vi "Leakage_Keithley6517A.vi"(5 "Number of Points":sgl=1.0 min=0 max=9999.9 step=0.1 format="%.1f", 6 "Interval(secs)":sgl=1.0 min=0 max=9999.9 step=0.1 format="%.1f", 7 "Bias Voltage":sgl=1.0 min=-1000 max=1000 step=0.1 format="%.1f", 8 "error in":T1, 11 "GPIB address":string="27") -> (0 "error out":T1, 3 "Test Data":sgl[][](array[numeric])=[[1.0, 2.2355776e-13]] format="%.6p")   [LabVIEW 2010]
doc: "This VI performs the Capacitor Leakage Test Sequence in the 6517A. \n\nParameters:\nGPIB Address: Default to 27\n\nBias Voltage\n-1000 to +1000\n\nBias Time:\n0 to 9999.9\n\nDischarge Time:\n0 to 9999.9"
panel:
  in  "control":sgl[](array[numeric]) format="%.2f"
  out "?":string="Current"
  # "KEITHLEY"
  # "6517A Capacitor Leakage Test"
  # "Voltage"
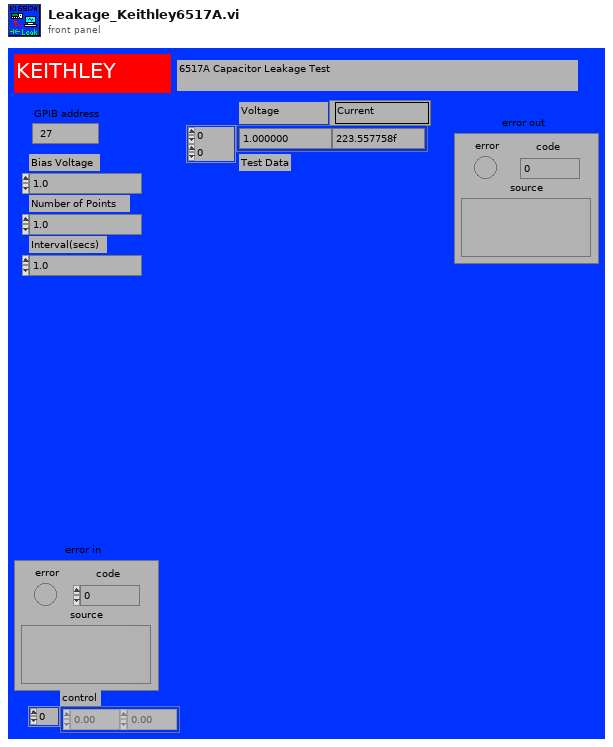
[diagram p1: front panel]
types:
  T1 = cluster{"error":bool, "code":i32, "source":string}
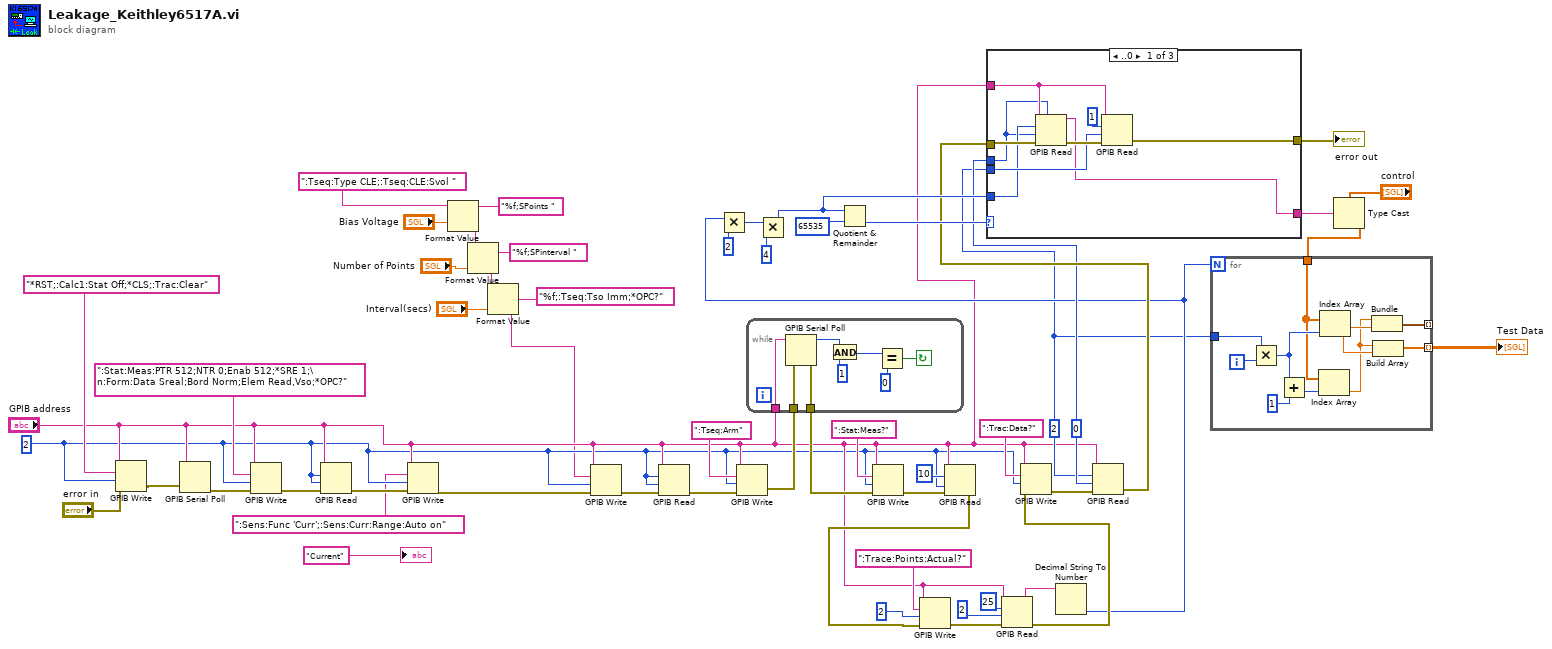
[diagram p0: block diagram]
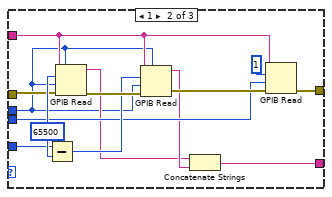
[diagram p2: hidden frame]
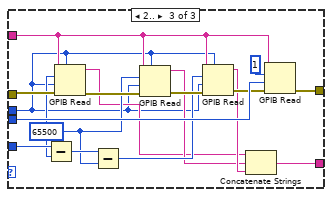
[diagram p3: hidden frame]
diagram:
  w27 = 0
  w12 = 2
  w4 = 2
  n1 = GPIB Write(0:"GPIB address", 1:"*RST;:Calc1:Stat Off;*CLS;:Trac:Clear", 2:w4, 3:"error in") -> (6:w53:errorcluster)  [unwired: 1 in, 1 out]
  n2 = GPIB Serial Poll(0:"GPIB address", 1:w53) -> (4:w52:errorcluster)  [unwired: 2 out]
  n3 = GPIB Write(0:"GPIB address", 1:":Stat:Meas:PTR 512;NTR 0;Enab 512;*SRE 1;\n:Form:Data Sreal;Bord Norm;Elem Read,Vso;*OPC?", 2:w4, 3:w52) -> (6:w50:errorcluster)  [unwired: 1 in, 1 out]
  n4 = GPIB Read(0:"GPIB address", 1:w4, 2:w4, 3:w50) -> (7:w6:errorcluster)  [unwired: 1 in, 2 out]
  n5 = GPIB Write(0:"GPIB address", 1:":Sens:Func 'Curr';:Sens:Curr:Range:Auto on", 2:w4, 3:w6) -> (6:w7:errorcluster)  [unwired: 1 in, 1 out]
  n6 = Format Value(string ("")=":Tseq:Type CLE;:Tseq:CLE:Svol ", format string="%f;SPoints ", value (0)="Bias Voltage") -> (output string=w47:string)
  n7 = Format Value(string ("")=w47, format string="%f;SPinterval ", value (0)="Number of Points") -> (output string=w45:string)
  n8 = Format Value(string ("")=w45, format string="%f;:Tseq:Tso Imm;*OPC?", value (0)="Interval(secs)") -> (output string=w1:string)
  n9 = GPIB Write(0:"GPIB address", 1:w1, 2:w4, 3:w7) -> (6:w43:errorcluster)  [unwired: 1 in, 1 out]
  n10 = GPIB Read(0:"GPIB address", 1:w4, 2:w4, 3:w43) -> (7:w42:errorcluster)  [unwired: 1 in, 2 out]
  n11 = GPIB Write(0:"GPIB address", 1:":Tseq:Arm", 2:w4, 3:w42) -> (6:w35:errorcluster)  [unwired: 1 in, 1 out]
  n12 = while {
    tunnel: w35 -> [w59]
    tunnel: [w58] -> w34
    tunnel: "GPIB address" -> [w57]
    stop <- w62 continue-if-true
    n13 = GPIB Serial Poll(0:w57, 1:w59) -> (2:w61:i16, 4:w58:errorcluster)  [unwired: 1 out]
    n14 = And(x=w61, y=1) -> (x .and. y?=w56:i32)
    n15 = Equal?(x=w56, y=0) -> (x = y?=w62:bool)
  }
  n16 = GPIB Write(0:"GPIB address", 1:":Stat:Meas?", 2:w4, 3:w34) -> (6:w39:errorcluster)  [unwired: 1 in, 1 out]
  n17 = GPIB Read(0:"GPIB address", 1:10, 2:w4, 3:w39) -> (7:w20:errorcluster)  [unwired: 1 in, 2 out]
  n18 = GPIB Write(0:"GPIB address", 1:":Trace:Points:Actual?", 2:2, 3:w20) -> (6:w23:errorcluster)  [unwired: 1 in, 1 out]
  n19 = GPIB Read(0:"GPIB address", 1:25, 2:2, 3:w23) -> (5:w18:string, 7:w19:errorcluster)  [unwired: 1 in, 1 out]
  n20 = GPIB Write(0:"GPIB address", 1:":Trac:Data?", 2:w4, 3:w19) -> (6:w36:errorcluster)  [unwired: 1 in, 1 out]
  n21 = Decimal String To Number(string=w18) -> (number=w13:i32)  [unwired: 2 in, 1 out]
  n22 = Multiply(x=w13, y=2) -> (x*y=w14:i32)
  n23 = Multiply(x=w14, y=4) -> (x*y=w30:i32)
  n24 = Quotient & Remainder(x=w30, y=65535) -> (floor(x/y)=w31:i32)  [unwired: 1 out]
  n25 = GPIB Read(0:"GPIB address", 1:w12, 2:w27, 3:w36) -> (7:w28:errorcluster)  [unwired: 1 in, 2 out]
  n26 = case shown="..0" w31 {
    tunnel: w28 -> [w70 w78 w100]
    tunnel: w12 -> [w69 w80 w102]
    tunnel: [w68 w77 w92] -> w11
    tunnel: [w67 w81 w101] -> w26
    tunnel: w30 -> [w66 w79 w98]
    tunnel: "GPIB address" -> [w65 w74 w88]
    tunnel: w27 -> [w64 w73 w87]
    frame ..0 {
      n27 = GPIB Read(0:w65, 1:w66, 2:w64, 3:w70, 4:w64) -> (5:w68:string, 7:w71:errorcluster)  [unwired: 1 out]
      n28 = GPIB Read(0:w65, 1:1, 2:w69, 3:w71) -> (7:w67:errorcluster)  [unwired: 1 in, 2 out]
    }
    frame 1 {
      w83 = 65500
      n29 = Subtract(x=w79, y=w83) -> (x-y=w82:i32)
      n30 = GPIB Read(0:w74, 1:w83, 2:w73, 3:w78, 4:w73) -> (5:w75:string, 7:w85:errorcluster)  [unwired: 1 out]
      n31 = GPIB Read(0:w74, 1:w82, 2:w73, 3:w85, 4:w73) -> (5:w76:string, 7:w84:errorcluster)  [unwired: 1 out]
      n32 = Concatenate Strings(w75, w76) -> (w77:string)
      n33 = GPIB Read(0:w74, 1:1, 2:w80, 3:w84) -> (7:w81:errorcluster)  [unwired: 1 in, 2 out]
    }
    frame 2.. {
      w94 = 65500
      n34 = Subtract(x=w98, y=w94) -> (x-y=w95:i32)
      n35 = GPIB Read(0:w88, 1:w94, 2:w87, 3:w100, 4:w87) -> (5:w89:string, 7:w99:errorcluster)  [unwired: 1 out]
      n36 = Subtract(x=w95, y=w94) -> (x-y=w93:i32)
      n37 = GPIB Read(0:w88, 1:w94, 2:w87, 3:w99, 4:w87) -> (5:w90:string, 7:w96:errorcluster)  [unwired: 1 out]
      n38 = GPIB Read(0:w88, 1:w93, 2:w87, 3:w96, 4:w87) -> (5:w91:string, 7:w97:errorcluster)  [unwired: 1 out]
      n39 = Concatenate Strings(w89, w90, w91) -> (w92:string)
      n40 = GPIB Read(0:w88, 1:1, 2:w102, 3:w97) -> (7:w101:errorcluster)  [unwired: 1 in, 2 out]
    }
  }
  "error out" <- w26
  n41 = Type Cast(type="control", x=w11) -> (*(type *) &x=w10:sgl[])
  n42 = for {
    N: w13 -> [_]
    tunnel: w12 -> [w112]
    tunnel: w10 -> [w108]
    tunnel: [w107] -> w8 mode=indexing
    tunnel: [w104] -> _ mode=indexing
    i -> [w111]
    n43 = Multiply(x=w112, y=w111) -> (x*y=w110:i32)
    n44 = Add(x=w110, y=1) -> (x+y=w109:i32)
    n45 = Index Array(array=w108, index=w109) -> (element=w105:sgl)
    n46 = Index Array(array=w108, index=w110) -> (element=w106:sgl)
    n47 = Bundle("Current"=w105, "Current"=w106) -> (w104:cluster{"Current":sgl, "Current":sgl})  [unwired: 1 in]
    n48 = Build Array(w105, w106) -> (w107:sgl[])
  }
  "Test Data" <- w8
  "?" <- "Current"
